vi "cursor window logic -- no plot.vi"(4 "h. offset":dbl, 6 "CursIdx":i32, 7 "cursor window action":T3=enum."check", 8 "window":dbl=nan, 9 "center":dbl=nan, 10 "cursor window in":refnum<vi>, 11 "cursor window init":T2={"left"=2378.60310421286, "right "=2421.6740576496672, "center"=2421.6740576496672, "window"=2421.6740576496672, "cursors"=[], "relative"=0, "absolute"=0, "fixed vertical offset"=2421.6740576496672, "vertical offset"=2421.6740576496672, "skew"=2421.6740576496672, "default window frac"=2421.6740576496672, "kind"=enum."skewed", "skew.left"=2421.6740576496672, "skew.right"=2421.6740576496672, "Plot ref"=refnum, "wing order"=enum."back"}) -> ()   [LabVIEW 2010]
uses:
  stack action -- control.ctl
  cursor window action.ctl
  cursor winow.ctl
  cursor winow control -- no plot.ctl
panel:
  out "cursor window out":T1={"left"=2378.60310421286, "right "=2421.6740576496672, "center"=2421.6740576496672, "window"=2421.6740576496672, "skew"=2421.6740576496672, "default window frac"=2421.6740576496672, "kind"=enum."skewed", "skew.left"=2421.6740576496672, "skew.right"=2421.6740576496672, "wing order"=enum."back"}
  in  "cursor window":T1={"left"=2378.60310421286, "right "=2421.6740576496672, "center"=2421.6740576496672, "window"=2421.6740576496672, "skew"=2421.6740576496672, "default window frac"=2421.6740576496672, "kind"=enum."skewed", "skew.left"=2421.6740576496672, "skew.right"=2421.6740576496672, "wing order"=enum."back"}
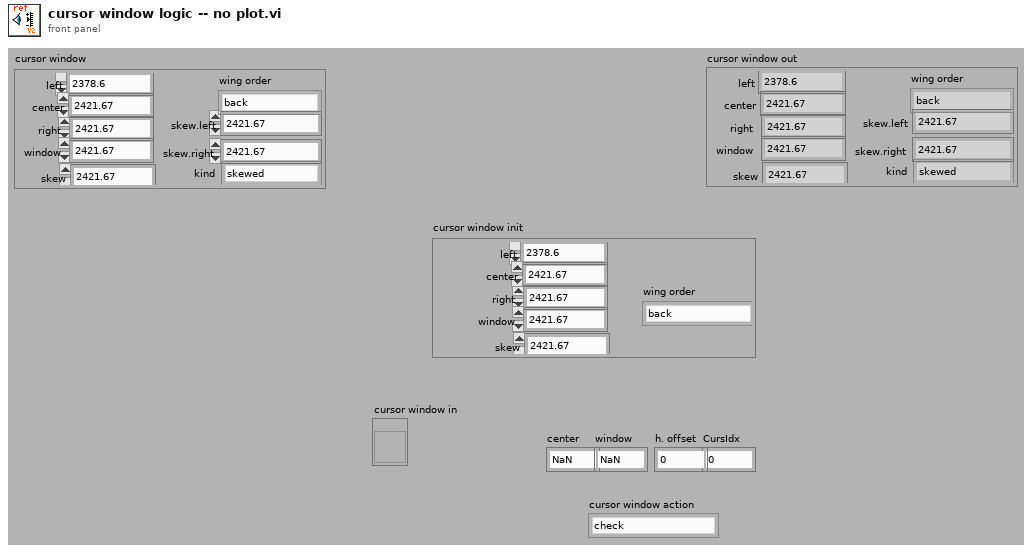
[diagram p1: front panel]
types:
  T1 = typedef "cursor winow control -- no plot.ctl" = cluster{"left":dbl, "right ":dbl, "center":dbl, "window":dbl, "skew":dbl, "default window frac":dbl, "kind":enum16{"symmetric", "skewed", "fancy"}, "skew.left":dbl, "skew.right":dbl, "wing order":enum16{"forw", "back"}}
  T2 = typedef "cursor winow.ctl" = cluster{"left":dbl, "right ":dbl, "center":dbl, "window":dbl, "cursors":i32[], "relative":i32, "absolute":i32, "fixed vertical offset":dbl, "vertical offset":dbl, "skew":dbl, "default window frac":dbl, "kind":enum16{"symmetric", "skewed", "fancy"}, "skew.left":dbl, "skew.right":dbl, "Plot ref":refnum<vi>, "wing order":enum16{"forw", "back"}}
  T3 = typedef "cursor window action.ctl" = enum16{"balance", "h. offset change", "cursor moves", "change center", "change window", "init", "check", "reset", "set y to middle", "idle", "-write all Y", "-write left.X", "-write center.X", "-write right.X", "-write all X", "-change center", "-change window", "-change skew", "-read cursor 2", "-read cursor 1", "-read cursor 0", "-read all cursors", "-reset", "-read plot scale", "-set y to middle", "-Q: center.Y is visible", "-Q: window is visible", "-parse center.Y", "-right left from center", "-left move", "-right move", "-set center.Y", "-empty", "-set cursors to default", "-check", "-write center.Y", "-copy cursor 1", "-copy cursor 0", "-copy cursor 2", "move right", "move left", "shrink", "broaden", "skew up", "skew down", "-write plot scale", "zoom X", "change cen&win"}
  T4 = typedef "stack action -- control.ctl" = enum16{"push", "pop", "check"}
  T5 = cluster{"center":dbl, "window":dbl, "h.offset":dbl, "cursor window":T2}
  T6 = cluster{"right.Y":dbl, "right.X":dbl, "left.X":dbl, "left.Y":dbl, "center.X":dbl, "center.Y":dbl, "scale.x.max":dbl, "scale.x.min":dbl, "scale.y.range":dbl, "scale.y.min":dbl, "scale.x.range":dbl, "scale.y.max":dbl, "skew":dbl, "cursor":i32, "scale.x.center":dbl, "scale.x.halfwidth":dbl, "scale.y.center":dbl, "scale.y.halfwidth":dbl}
  T7 = cluster{"left":dbl, "right ":dbl, "center":dbl, "window":dbl, "cursors":i32[], "relative":i32, "absolute":i32, "fixed vertical offset":dbl, "vertical offset":dbl, "skew":dbl, "default window frac":dbl, "kind":enum16{"symmetric", "skewed", "fancy"}, "skew.left":dbl, "skew.right":dbl, "Plot ref":refnum<vi>, "wing order":enum16{"forw", "back"}}
  T8 = typedef "comparison control.ctl" = enum16{"not a number", "above", "in range", "below"}
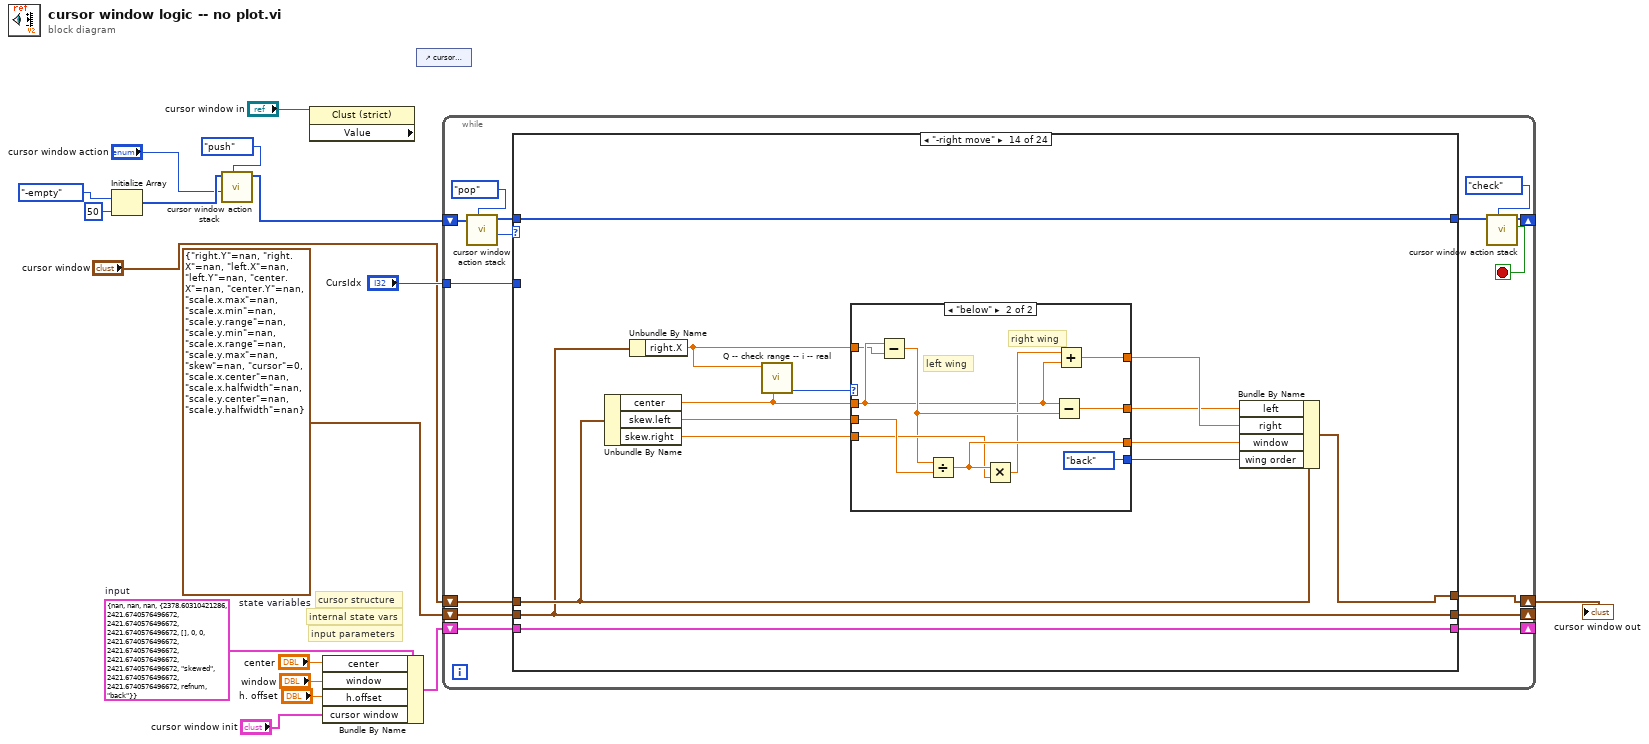
[diagram p0: block diagram]
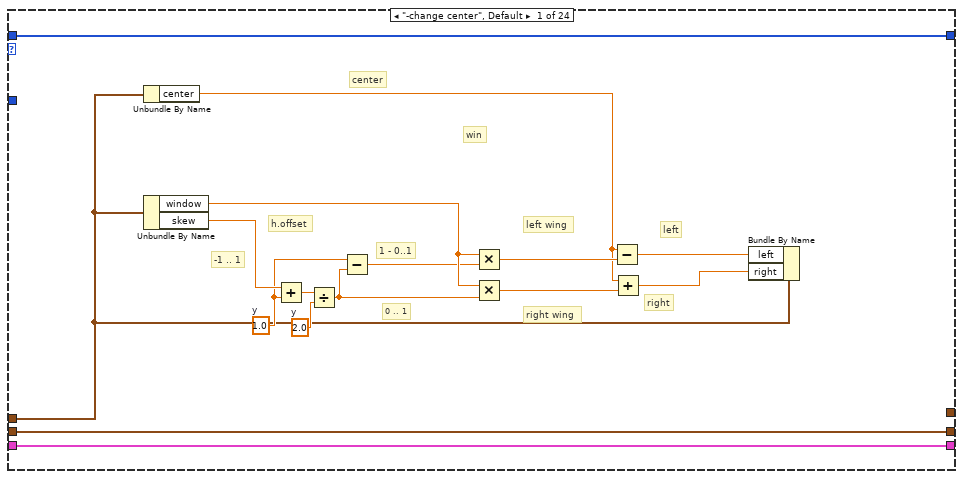
[diagram p2: hidden frame]
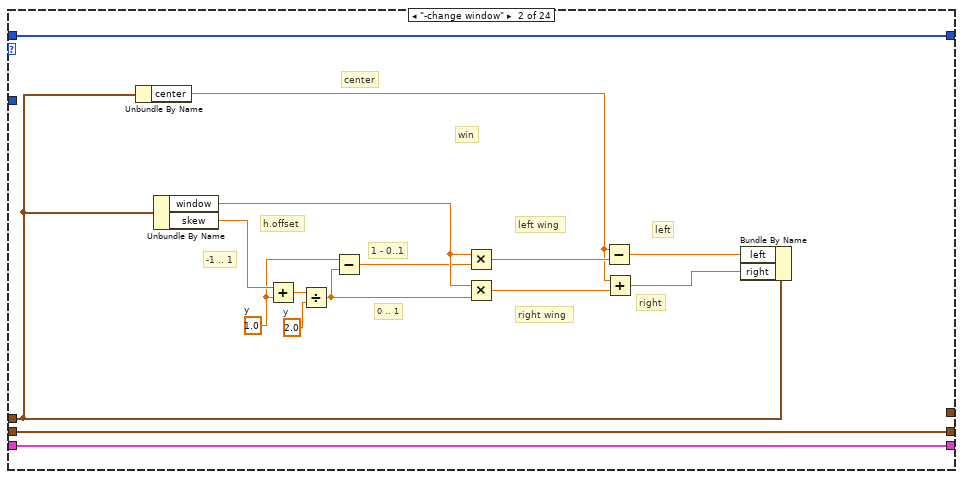
[diagram p3: hidden frame]
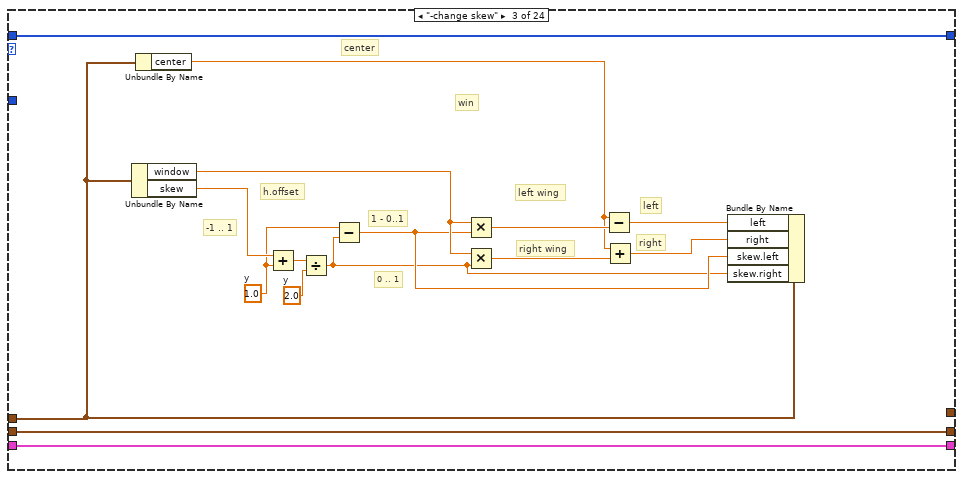
[diagram p4: hidden frame]
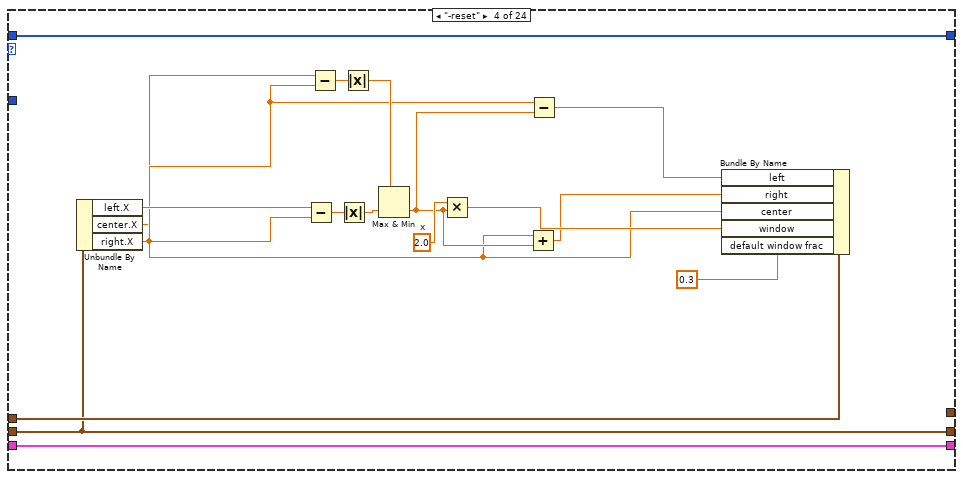
[diagram p5: hidden frame]
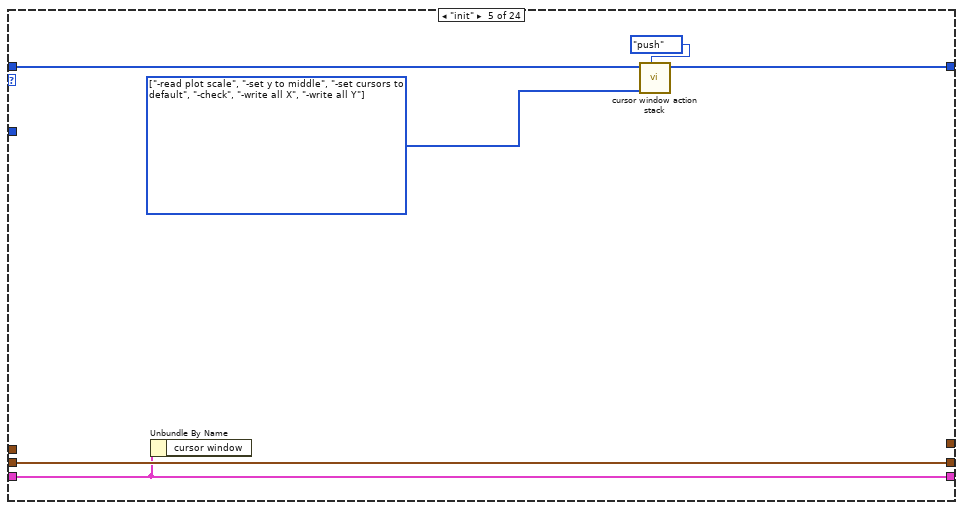
[diagram p6: hidden frame]
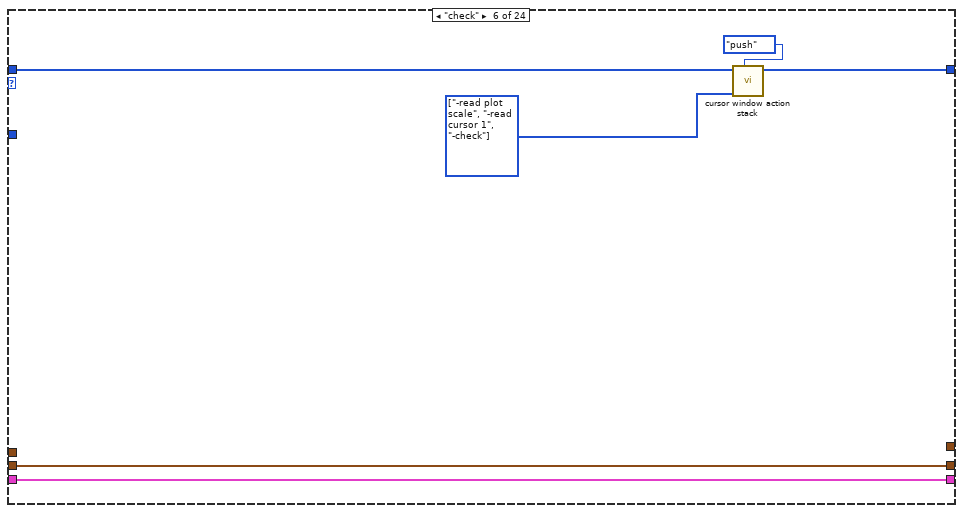
[diagram p7: hidden frame]
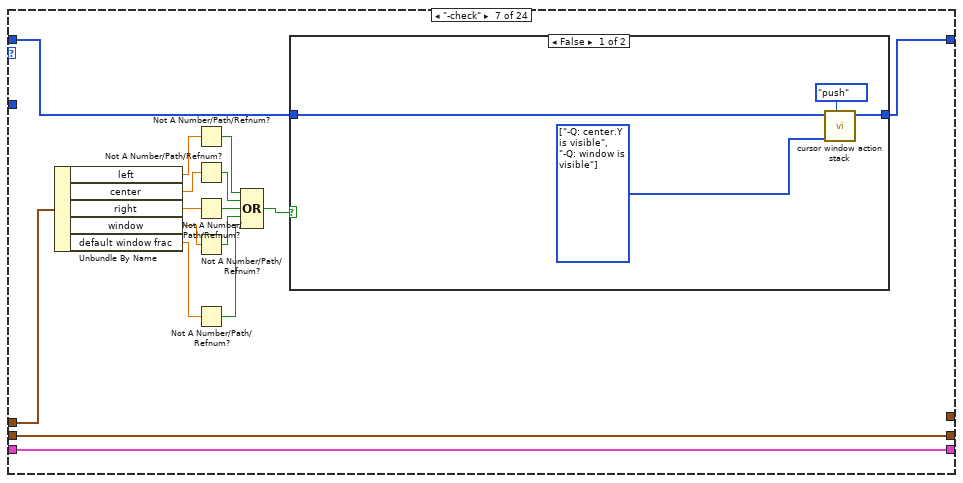
[diagram p8: hidden frame]
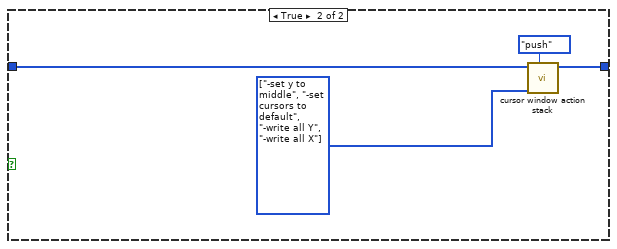
[diagram p9: hidden frame]
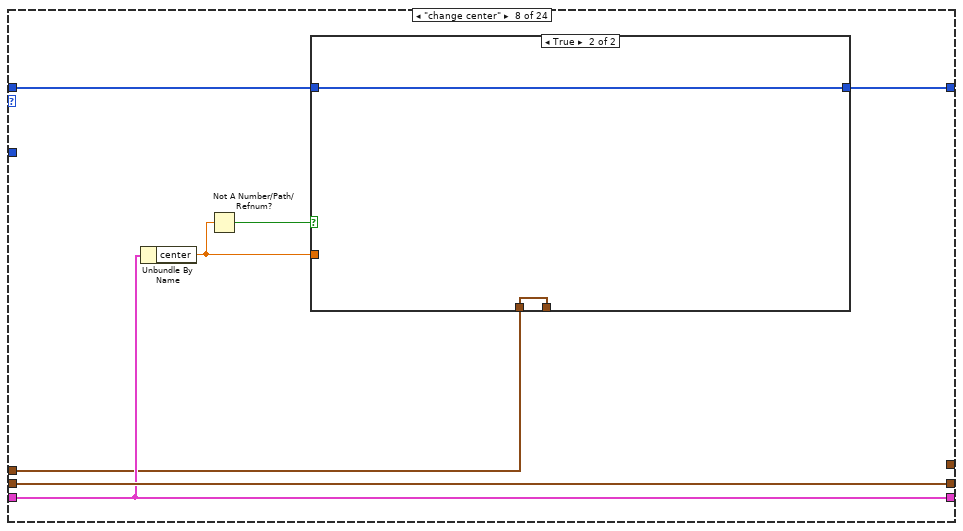
[diagram p10: hidden frame]
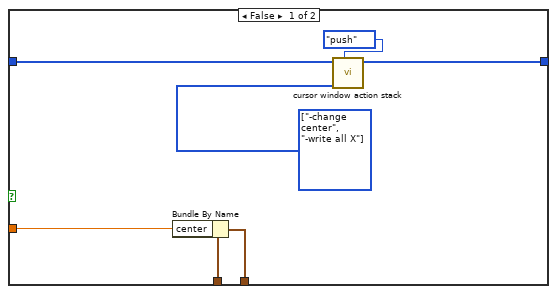
[diagram p11: hidden frame]
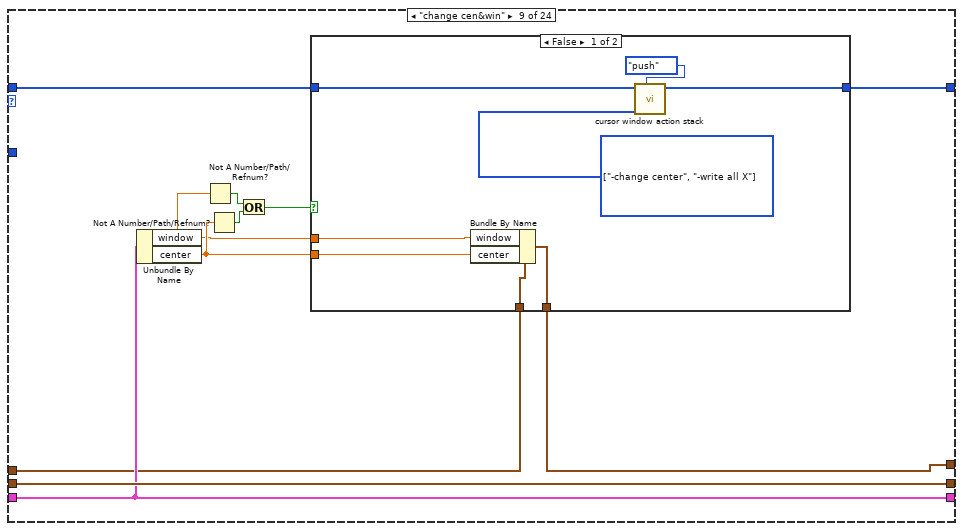
[diagram p12: hidden frame]
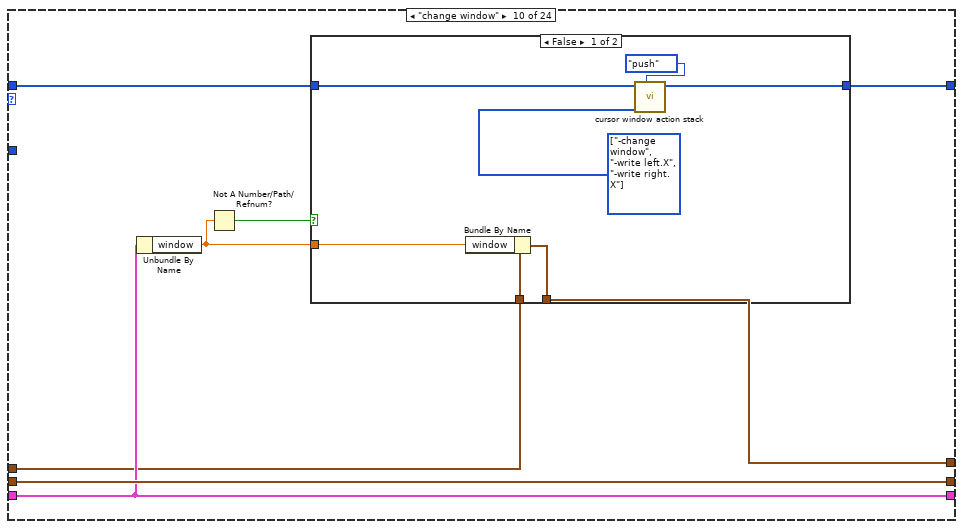
[diagram p14: hidden frame]
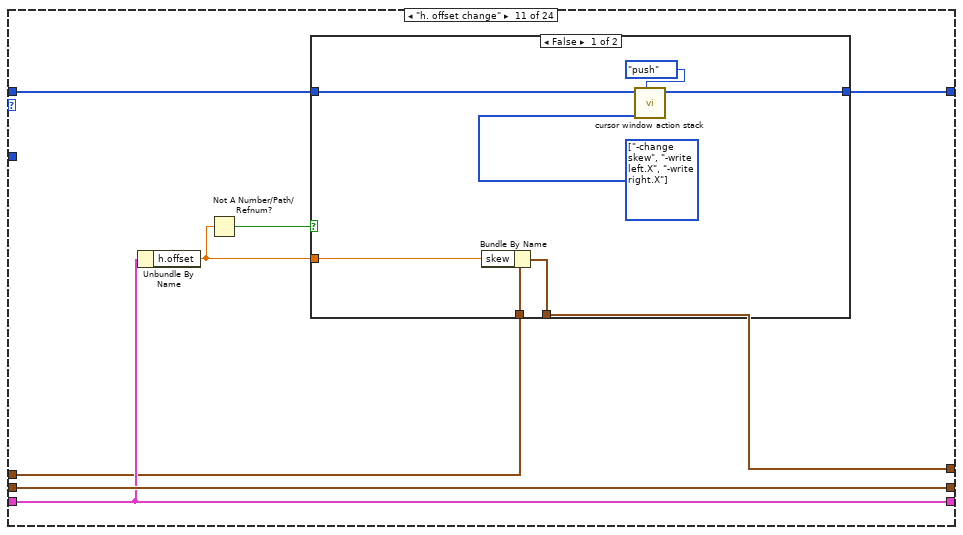
[diagram p16: hidden frame]
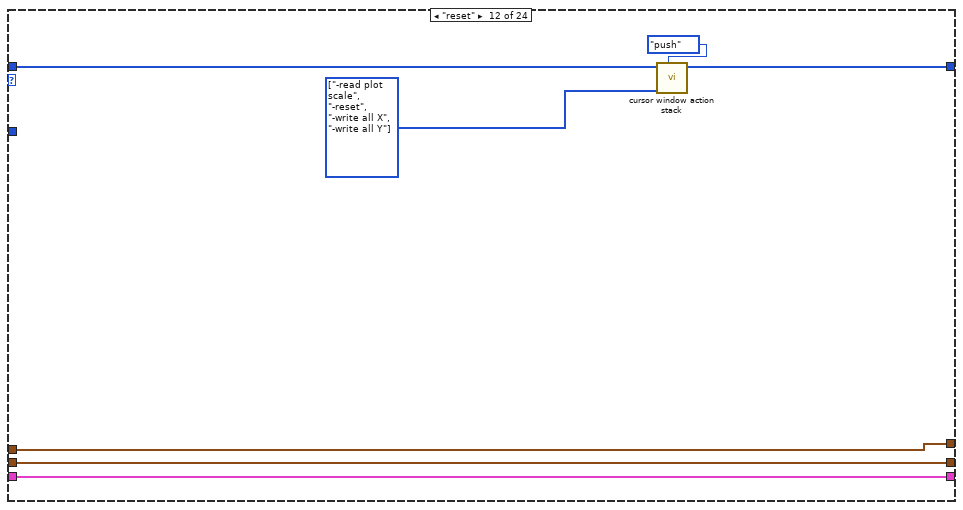
[diagram p18: hidden frame]
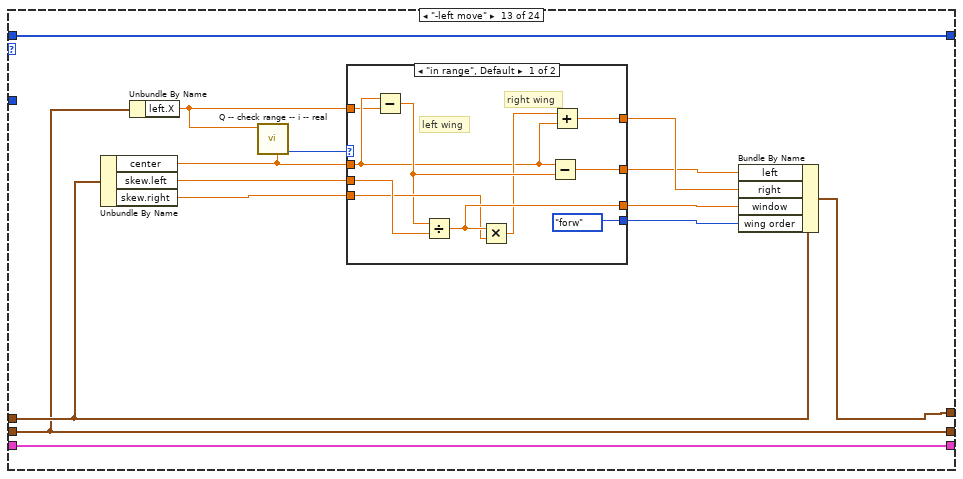
[diagram p19: hidden frame]
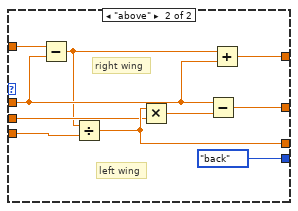
[diagram p20: hidden frame]
diagram:
  w17 = T5 {"center"=nan, "window"=nan, "h.offset"=nan, "cursor window"={"left"=2378.60310421286, "right "=2421.6740576496672, "center"=2421.6740576496672, "window"=2421.6740576496672, "cursors"=[], "relative"=0, "absolute"=0, "fixed vertical offset"=2421.6740576496672, "vertical offset"=2421.6740576496672, "skew"=2421.6740576496672, "default window frac"=2421.6740576496672, "kind"=enum."skewed", "skew.left"=2421.6740576496672, "skew.right"=2421.6740576496672, "Plot ref"=refnum, "wing order"=enum."back"}}  # input
  w18 = T6 {"right.Y"=nan, "right.X"=nan, "left.X"=nan, "left.Y"=nan, "center.X"=nan, "center.Y"=nan, "scale.x.max"=nan, "scale.x.min"=nan, "scale.y.range"=nan, "scale.y.min"=nan, "scale.x.range"=nan, "scale.y.max"=nan, "skew"=nan, "cursor"=0, "scale.x.center"=nan, "scale.x.halfwidth"=nan, "scale.y.center"=nan, "scale.y.halfwidth"=nan}  # state variables
  # "input parameters"
  # "internal state vars"
  # "cursor structure"
  n1 = Initialize Array(cursor_window_action."-empty" ("cursor window action"), 50 ("dimension size")) -> (w6:T3[])
  n2 = call "cursor window action stack.vi"("stack action"=stack_action_--_control."push", "cursor window action"="cursor window action", "command stack"=w6) -> ("command stack out"=w5:T3[])  [unwired: 6 in, 2 out]
  n3 = property class="Clust (strict)"(reference="cursor window in") -> (reference out=w19:refnum<vi>, "Value"=w11:T7)  [unwired: 1 in, 1 out]
  n4 = Bundle By Name(cluster=w17, "center"="center", "window"="window", "h.offset"="h. offset", "cursor window"="cursor window init") -> (w13:T5)
  n5 = control-ref of="cursor window init"() -> ()  [unwired: 1 out]
  n6 = while {
    shift-right: [w27] -> _
    shift-left: w5 -> [w33]
    shift-right: [w20] -> w1
    shift-left: "cursor window" -> [w34]
    shift-right: [w24] -> _
    shift-left: w13 -> [w25]
    shift-right: [w22] -> _
    shift-left: w18 -> [w23]
    tunnel: "CursIdx" -> [w21]
    stop <- w26 stop-if-true
    n7 = call "cursor window action stack.vi"("stack action"=stack_action_--_control."pop", "command stack"=w33) -> ("cursor window action out"=w32:T3, "command stack out"=w30:T3[])  [unwired: 7 in, 1 out]
    n8 = case shown="\"-right move\"" w32 {
      tunnel: w34 -> [w36 w53 w72 w94 _ w111 w121 w143 w164 w181 w198 w214 w231 w265 w291 w302 w315 w329 w335 w355 w361 w374 w395 w419]
      tunnel: [w40 w57 w76 w93 w105 w114 w118 w148 w168 w186 w203 w217 w228 w262 w292 w300 w320 w330 w343 w356 w370 w378 w399 w421] -> w28
      tunnel: w30 -> [w40 w57 w76 w93 w106 w115 w119 w147 w167 w185 w202 w218 w228 w262 w292 w300 w320 w331 w344 w357 w371 w379 w400 w422]
      tunnel: w25 -> [w37 w54 w73 w92 w109 w112 w122 w146 w166 w184 w201 w220 w230 w264 w289 w303 w319 w325 w341 w351 w368 w375 w396 w426]
      tunnel: [w37 w54 w73 w92 w109 w112 w122 w146 w166 w184 w201 w220 w230 w264 w289 w303 w319 w325 w341 w351 w368 w375 w396 w426] -> w24
      tunnel: w23 -> [w39 w56 w75 w91 w110 w113 w123 w149 w169 w187 w204 w219 w229 w263 w290 w305 w318 w326 w342 w352 w369 w376 w397 w425]
      tunnel: [w39 w56 w75 w91 w110 w113 w123 w149 w169 w187 w204 w219 w229 w263 w290 w305 w318 w326 w342 w352 w369 w376 w397 w425] -> w22
      tunnel: w21 -> [_ _ _ _ _ _ _ _ _ _ _ _ _ _ _ _ _ _ _ _ _ _ _ _]
      tunnel: [_ _ _ _ _ _ _ _ w159 w180 w197 w214 w221 w255 _ _ _ _ _ _ _ _ _ _] -> w20
      frame "-change center", Default {
        w45 = 1.0  # y
        w47 = 2.0  # y
        # "1 - 0..1"
        # "right"
        # "left"
        # "win"
        # "h.offset"
        # "center"
        # "left wing"
        # "right wing"
        # "0 .. 1"
        # "-1 .. 1"
        n9 = Unbundle By Name(w36) -> ("center"=w38:dbl)
        n10 = Unbundle By Name(w36) -> ("window"=w50:dbl, "skew"=w51:dbl)
        n11 = Add(x=w51, y=w45) -> (x+y=w46:dbl)
        n12 = Divide(x=w46, y=w47) -> (x/y=w42:dbl)
        n13 = Subtract(x=w45, y=w42) -> (x-y=w41:dbl)
        n14 = Multiply(x=w50, y=w41) -> (x*y=w44:dbl)
        n15 = Multiply(x=w50, y=w42) -> (x*y=w43:dbl)
        n16 = Subtract(x=w38, y=w44) -> (x-y=w49:dbl)
        n17 = Add(x=w38, y=w43) -> (x+y=w48:dbl)
        n18 = Bundle By Name(cluster=w36, "left"=w49, "right"=w48) -> (w35:T1)
      }
      frame "-change window" {
        w62 = 1.0  # y
        w64 = 2.0  # y
        # "1 - 0..1"
        # "right"
        # "left"
        # "win"
        # "h.offset"
        # "center"
        # "left wing"
        # "right wing"
        # "0 .. 1"
        # "-1 .. 1"
        n19 = Unbundle By Name(w53) -> ("center"=w55:dbl)
        n20 = Unbundle By Name(w53) -> ("window"=w67:dbl, "skew"=w68:dbl)
        n21 = Add(x=w68, y=w62) -> (x+y=w63:dbl)
        n22 = Divide(x=w63, y=w64) -> (x/y=w59:dbl)
        n23 = Subtract(x=w62, y=w59) -> (x-y=w58:dbl)
        n24 = Multiply(x=w67, y=w58) -> (x*y=w61:dbl)
        n25 = Multiply(x=w67, y=w59) -> (x*y=w60:dbl)
        n26 = Subtract(x=w55, y=w61) -> (x-y=w66:dbl)
        n27 = Add(x=w55, y=w60) -> (x+y=w65:dbl)
        n28 = Bundle By Name(cluster=w53, "left"=w66, "right"=w65) -> (w52:T1)
      }
      frame "-change skew" {
        w79 = 1.0  # y
        w81 = 2.0  # y
        # "1 - 0..1"
        # "right"
        # "left"
        # "win"
        # "h.offset"
        # "center"
        # "left wing"
        # "right wing"
        # "0 .. 1"
        # "-1 .. 1"
        n29 = Unbundle By Name(w72) -> ("window"=w84:dbl, "skew"=w85:dbl)
        n30 = Unbundle By Name(w72) -> ("center"=w74:dbl)
        n31 = Add(x=w85, y=w79) -> (x+y=w80:dbl)
        n32 = Divide(x=w80, y=w81) -> (x/y=w70:dbl)
        n33 = Subtract(x=w79, y=w70) -> (x-y=w71:dbl)
        n34 = Multiply(x=w84, y=w71) -> (x*y=w78:dbl)
        n35 = Multiply(x=w84, y=w70) -> (x*y=w77:dbl)
        n36 = Subtract(x=w74, y=w78) -> (x-y=w83:dbl)
        n37 = Add(x=w74, y=w77) -> (x+y=w82:dbl)
        n38 = Bundle By Name(cluster=w72, "left"=w83, "right"=w82, "skew.left"=w71, "skew.right"=w70) -> (w69:T1)
      }
      frame "-reset" {
        w99 = 2.0  # x
        n39 = Unbundle By Name(w91) -> ("left.X"=w90:dbl, "center.X"=w88:dbl, "right.X"=w89:dbl)
        n40 = Subtract(x=w90, y=w89) -> (x-y=w102:dbl)
        n41 = Subtract(x=w88, y=w89) -> (x-y=w103:dbl)
        n42 = Absolute Value(x=w102) -> (abs(x)=w100:dbl)
        n43 = Absolute Value(x=w103) -> (abs(x)=w101:dbl)
        n44 = Max & Min(x=w101, y=w100) -> (min(x,y)=w97:dbl)  [unwired: 1 out]
        n45 = Multiply(x=w99, y=w97) -> (x*y=w98:dbl)
        n46 = Add(x=w89, y=w97) -> (x+y=w95:dbl)
        n47 = Subtract(x=w89, y=w97) -> (x-y=w96:dbl)
        n48 = Bundle By Name(cluster=w94, "left"=w96, "right"=w95, "center"=w89, "window"=w98, "default window frac"=0.3) -> (w87:T1)
      }
      frame "init" {
        w107 = T3[] [enum."-read plot scale", enum."-set y to middle", enum."-set cursors to default", enum."-check", enum."-write all X", enum."-write all Y"] items=["balance", "h. offset change", "cursor moves", "change center", "change window", "init", "check", "reset", "set y to middle", "idle", "-write all Y", "-write left.X", "-write center.X", "-write right.X", "-write all X", "-change center", "-change window", "-change skew", "-read cursor 2", "-read cursor 1", "-read cursor 0", "-read all cursors", "-reset", "-read plot scale", "-set y to middle", "-Q: center.Y is visible", "-Q: window is visible", "-parse center.Y", "-right left from center", "-left move", "-right move", "-set center.Y", "-empty", "-set cursors to default", "-check", "-write center.Y", "-copy cursor 1", "-copy cursor 0", "-copy cursor 2", "move right", "move left", "shrink", "broaden", "skew up", "skew down", "-write plot scale", "zoom X", "change cen&win"]
        n49 = Unbundle By Name(w109) -> ("cursor window"=w104:T2)
        n50 = call "cursor window action stack.vi"("stack action"=stack_action_--_control."push", "action list"=w107, "command stack"=w106) -> ("command stack out"=w105:T3[])  [unwired: 6 in, 2 out]
      }
      frame "check" {
        w116 = T3[] [enum."-read plot scale", enum."-read cursor 1", enum."-check"] items=["balance", "h. offset change", "cursor moves", "change center", "change window", "init", "check", "reset", "set y to middle", "idle", "-write all Y", "-write left.X", "-write center.X", "-write right.X", "-write all X", "-change center", "-change window", "-change skew", "-read cursor 2", "-read cursor 1", "-read cursor 0", "-read all cursors", "-reset", "-read plot scale", "-set y to middle", "-Q: center.Y is visible", "-Q: window is visible", "-parse center.Y", "-right left from center", "-left move", "-right move", "-set center.Y", "-empty", "-set cursors to default", "-check", "-write center.Y", "-copy cursor 1", "-copy cursor 0", "-copy cursor 2", "move right", "move left", "shrink", "broaden", "skew up", "skew down", "-write plot scale", "zoom X", "change cen&win"]
        n51 = call "cursor window action stack.vi"("stack action"=stack_action_--_control."push", "action list"=w116, "command stack"=w115) -> ("command stack out"=w114:T3[])  [unwired: 6 in, 2 out]
      }
      frame "-check" {
        n52 = Unbundle By Name(w121) -> ("left"=w131:dbl, "center"=w130:dbl, "right"=w132:dbl, "window"=w133:dbl, "default window frac"=w125:dbl)
        n53 = Not A Number/Path/Refnum?(number/path/refnum=w131) -> (NaN/Path/Refnum?=w129:bool)
        n54 = Not A Number/Path/Refnum?(number/path/refnum=w130) -> (NaN/Path/Refnum?=w128:bool)
        n55 = Not A Number/Path/Refnum?(number/path/refnum=w132) -> (NaN/Path/Refnum?=w127:bool)
        n56 = Not A Number/Path/Refnum?(number/path/refnum=w133) -> (NaN/Path/Refnum?=w126:bool)
        n57 = Not A Number/Path/Refnum?(number/path/refnum=w125) -> (NaN/Path/Refnum?=w124:bool)
        n58 = Compound Arithmetic op=OR(w129, w128, w127, w126, w124) -> (w120:bool)
        n59 = case shown="False" w120 {
          tunnel: w119 -> [w135 w139]
          tunnel: [w134 w138] -> w118
          frame False {
            w136 = T3[] [enum."-Q: center.Y is visible", enum."-Q: window is visible"] items=["balance", "h. offset change", "cursor moves", "change center", "change window", "init", "check", "reset", "set y to middle", "idle", "-write all Y", "-write left.X", "-write center.X", "-write right.X", "-write all X", "-change center", "-change window", "-change skew", "-read cursor 2", "-read cursor 1", "-read cursor 0", "-read all cursors", "-reset", "-read plot scale", "-set y to middle", "-Q: center.Y is visible", "-Q: window is visible", "-parse center.Y", "-right left from center", "-left move", "-right move", "-set center.Y", "-empty", "-set cursors to default", "-check", "-write center.Y", "-copy cursor 1", "-copy cursor 0", "-copy cursor 2", "move right", "move left", "shrink", "broaden", "skew up", "skew down", "-write plot scale", "zoom X", "change cen&win"]
            n60 = call "cursor window action stack.vi"("stack action"=stack_action_--_control."push", "action list"=w136, "command stack"=w135) -> ("command stack out"=w134:T3[])  [unwired: 6 in, 2 out]
          }
          frame True {
            w140 = T3[] [enum."-set y to middle", enum."-set cursors to default", enum."-write all Y", enum."-write all X"] items=["balance", "h. offset change", "cursor moves", "change center", "change window", "init", "check", "reset", "set y to middle", "idle", "-write all Y", "-write left.X", "-write center.X", "-write right.X", "-write all X", "-change center", "-change window", "-change skew", "-read cursor 2", "-read cursor 1", "-read cursor 0", "-read all cursors", "-reset", "-read plot scale", "-set y to middle", "-Q: center.Y is visible", "-Q: window is visible", "-parse center.Y", "-right left from center", "-left move", "-right move", "-set center.Y", "-empty", "-set cursors to default", "-check", "-write center.Y", "-copy cursor 1", "-copy cursor 0", "-copy cursor 2", "move right", "move left", "shrink", "broaden", "skew up", "skew down", "-write plot scale", "zoom X", "change cen&win"]
            n61 = call "cursor window action stack.vi"("stack action"=stack_action_--_control."push", "action list"=w140, "command stack"=w139) -> ("command stack out"=w138:T3[])  [unwired: 6 in, 2 out]
          }
        }
      }
      frame "change center" {
        n62 = Unbundle By Name(w146) -> ("center"=w144:dbl)
        n63 = Not A Number/Path/Refnum?(number/path/refnum=w144) -> (NaN/Path/Refnum?=w145:bool)
        n64 = case shown="True" w145 {
          tunnel: [w156 w157] -> w148
          tunnel: w147 -> [w155 w157]
          tunnel: w143 -> [w152 w158]
          tunnel: w144 -> [w151 _]
          tunnel: [w150 w158] -> w142
          frame False {
            w153 = T3[] [enum."-change center", enum."-write all X"] items=["balance", "h. offset change", "cursor moves", "change center", "change window", "init", "check", "reset", "set y to middle", "idle", "-write all Y", "-write left.X", "-write center.X", "-write right.X", "-write all X", "-change center", "-change window", "-change skew", "-read cursor 2", "-read cursor 1", "-read cursor 0", "-read all cursors", "-reset", "-read plot scale", "-set y to middle", "-Q: center.Y is visible", "-Q: window is visible", "-parse center.Y", "-right left from center", "-left move", "-right move", "-set center.Y", "-empty", "-set cursors to default", "-check", "-write center.Y", "-copy cursor 1", "-copy cursor 0", "-copy cursor 2", "move right", "move left", "shrink", "broaden", "skew up", "skew down", "-write plot scale", "zoom X", "change cen&win"]
            n65 = Bundle By Name(cluster=w152, "center"=w151) -> (w150:T1)
            n66 = call "cursor window action stack.vi"("stack action"=stack_action_--_control."push", "action list"=w153, "command stack"=w155) -> ("command stack out"=w156:T3[])  [unwired: 6 in, 2 out]
          }
          frame True {
          }
        }
      }
      frame "change cen&win" {
        n67 = Unbundle By Name(w166) -> ("window"=w160:dbl, "center"=w165:dbl)
        n68 = Not A Number/Path/Refnum?(number/path/refnum=w160) -> (NaN/Path/Refnum?=w163:bool)
        n69 = Not A Number/Path/Refnum?(number/path/refnum=w165) -> (NaN/Path/Refnum?=w162:bool)
        n70 = Or(x=w163, y=w162) -> (x .or. y?=w161:bool)
        n71 = case shown="False" w161 {
          tunnel: [w177 w178] -> w168
          tunnel: w167 -> [w176 w178]
          tunnel: w164 -> [w173 w179]
          tunnel: w165 -> [w172 _]
          tunnel: [w171 w179] -> w159
          tunnel: w160 -> [w170 _]
          frame False {
            w174 = T3[] [enum."-change center", enum."-write all X"] items=["balance", "h. offset change", "cursor moves", "change center", "change window", "init", "check", "reset", "set y to middle", "idle", "-write all Y", "-write left.X", "-write center.X", "-write right.X", "-write all X", "-change center", "-change window", "-change skew", "-read cursor 2", "-read cursor 1", "-read cursor 0", "-read all cursors", "-reset", "-read plot scale", "-set y to middle", "-Q: center.Y is visible", "-Q: window is visible", "-parse center.Y", "-right left from center", "-left move", "-right move", "-set center.Y", "-empty", "-set cursors to default", "-check", "-write center.Y", "-copy cursor 1", "-copy cursor 0", "-copy cursor 2", "move right", "move left", "shrink", "broaden", "skew up", "skew down", "-write plot scale", "zoom X", "change cen&win"]
            n72 = Bundle By Name(cluster=w173, "window"=w170, "center"=w172) -> (w171:T1)
            n73 = call "cursor window action stack.vi"("stack action"=stack_action_--_control."push", "action list"=w174, "command stack"=w176) -> ("command stack out"=w177:T3[])  [unwired: 6 in, 2 out]
          }
          frame True {
          }
        }
      }
      frame "change window" {
        n74 = Unbundle By Name(w184) -> ("window"=w182:dbl)
        n75 = Not A Number/Path/Refnum?(number/path/refnum=w182) -> (NaN/Path/Refnum?=w183:bool)
        n76 = case shown="False" w183 {
          tunnel: [w194 w195] -> w186
          tunnel: w185 -> [w193 w195]
          tunnel: w181 -> [w190 w196]
          tunnel: w182 -> [w189 _]
          tunnel: [w188 w196] -> w180
          frame False {
            w191 = T3[] [enum."-change window", enum."-write left.X", enum."-write right.X"] items=["balance", "h. offset change", "cursor moves", "change center", "change window", "init", "check", "reset", "set y to middle", "idle", "-write all Y", "-write left.X", "-write center.X", "-write right.X", "-write all X", "-change center", "-change window", "-change skew", "-read cursor 2", "-read cursor 1", "-read cursor 0", "-read all cursors", "-reset", "-read plot scale", "-set y to middle", "-Q: center.Y is visible", "-Q: window is visible", "-parse center.Y", "-right left from center", "-left move", "-right move", "-set center.Y", "-empty", "-set cursors to default", "-check", "-write center.Y", "-copy cursor 1", "-copy cursor 0", "-copy cursor 2", "move right", "move left", "shrink", "broaden", "skew up", "skew down", "-write plot scale", "zoom X", "change cen&win"]
            n77 = Bundle By Name(cluster=w190, "window"=w189) -> (w188:T1)
            n78 = call "cursor window action stack.vi"("stack action"=stack_action_--_control."push", "action list"=w191, "command stack"=w193) -> ("command stack out"=w194:T3[])  [unwired: 6 in, 2 out]
          }
          frame True {
          }
        }
      }
      frame "h. offset change" {
        n79 = Unbundle By Name(w201) -> ("h.offset"=w199:dbl)
        n80 = Not A Number/Path/Refnum?(number/path/refnum=w199) -> (NaN/Path/Refnum?=w200:bool)
        n81 = case shown="False" w200 {
          tunnel: [w211 w212] -> w203
          tunnel: w202 -> [w210 w212]
          tunnel: w198 -> [w207 w213]
          tunnel: w199 -> [w206 _]
          tunnel: [w205 w213] -> w197
          frame False {
            w208 = T3[] [enum."-change skew", enum."-write left.X", enum."-write right.X"] items=["balance", "h. offset change", "cursor moves", "change center", "change window", "init", "check", "reset", "set y to middle", "idle", "-write all Y", "-write left.X", "-write center.X", "-write right.X", "-write all X", "-change center", "-change window", "-change skew", "-read cursor 2", "-read cursor 1", "-read cursor 0", "-read all cursors", "-reset", "-read plot scale", "-set y to middle", "-Q: center.Y is visible", "-Q: window is visible", "-parse center.Y", "-right left from center", "-left move", "-right move", "-set center.Y", "-empty", "-set cursors to default", "-check", "-write center.Y", "-copy cursor 1", "-copy cursor 0", "-copy cursor 2", "move right", "move left", "shrink", "broaden", "skew up", "skew down", "-write plot scale", "zoom X", "change cen&win"]
            n82 = Bundle By Name(cluster=w207, "skew"=w206) -> (w205:T1)
            n83 = call "cursor window action stack.vi"("stack action"=stack_action_--_control."push", "action list"=w208, "command stack"=w210) -> ("command stack out"=w211:T3[])  [unwired: 6 in, 2 out]
          }
          frame True {
          }
        }
      }
      frame "reset" {
        w215 = T3[] [enum."-read plot scale", enum."-reset", enum."-write all X", enum."-write all Y"] items=["balance", "h. offset change", "cursor moves", "change center", "change window", "init", "check", "reset", "set y to middle", "idle", "-write all Y", "-write left.X", "-write center.X", "-write right.X", "-write all X", "-change center", "-change window", "-change skew", "-read cursor 2", "-read cursor 1", "-read cursor 0", "-read all cursors", "-reset", "-read plot scale", "-set y to middle", "-Q: center.Y is visible", "-Q: window is visible", "-parse center.Y", "-right left from center", "-left move", "-right move", "-set center.Y", "-empty", "-set cursors to default", "-check", "-write center.Y", "-copy cursor 1", "-copy cursor 0", "-copy cursor 2", "move right", "move left", "shrink", "broaden", "skew up", "skew down", "-write plot scale", "zoom X", "change cen&win"]
        n84 = call "cursor window action stack.vi"("stack action"=stack_action_--_control."push", "action list"=w215, "command stack"=w218) -> ("command stack out"=w217:T3[])  [unwired: 6 in, 2 out]
      }
      frame "-left move" {
        n85 = Unbundle By Name(w231) -> ("center"=w224:dbl, "skew.left"=w227:dbl, "skew.right"=w226:dbl)
        n86 = Unbundle By Name(w229) -> ("left.X"=w225:dbl)
        n87 = call "Q -- check range -- i -- real.vi"("upper"=w224, "number"=w225) -> ("selector"=w223:T8)  [unwired: 7 in, 2 out]
        n88 = case shown="\"in range\", Default" w223 {
          tunnel: w225 -> [w236 w254]
          tunnel: w226 -> [w242 w253]
          tunnel: [w243 w252] -> w232
          tunnel: [w238 w247] -> w234
          tunnel: w227 -> [w244 w251]
          tunnel: [w240 w246] -> w233
          tunnel: w224 -> [w237 w250]
          tunnel: [enum16{"forw", "back"}."forw" ("wing order") enum16{"forw", "back"}."back" ("wing order")] -> w222
          frame "in range", Default {
            # "right wing"
            # "left wing"
            n89 = Subtract(x=w237, y=w236) -> (x-y=w241:dbl)
            n90 = Divide(x=w241, y=w244) -> (x/y=w243:dbl)
            n91 = Multiply(x=w243, y=w242) -> (x*y=w239:dbl)
            n92 = Subtract(x=w237, y=w241) -> (x-y=w240:dbl)
            n93 = Add(x=w239, y=w237) -> (x+y=w238:dbl)
          }
          frame "above" {
            # "right wing"
            # "left wing"
            n94 = Subtract(x=w254, y=w250) -> (x-y=w249:dbl)
            n95 = Divide(x=w249, y=w253) -> (x/y=w252:dbl)
            n96 = Multiply(x=w252, y=w251) -> (x*y=w248:dbl)
            n97 = Subtract(x=w250, y=w248) -> (x-y=w246:dbl)
            n98 = Add(x=w249, y=w250) -> (x+y=w247:dbl)
          }
        }
        n99 = Bundle By Name(cluster=w231, "left"=w233, "right"=w234, "window"=w232, "wing order"=w222) -> (w221:T1)
      }
      frame "-right move" {
        n100 = Unbundle By Name(w265) -> ("center"=w256:dbl, "skew.left"=w261:dbl, "skew.right"=w260:dbl)
        n101 = Unbundle By Name(w263) -> ("right.X"=w259:dbl)
        n102 = call "Q -- check range -- i -- real.vi"("lower"=w256, "number"=w259) -> ("selector"=w258:T8)  [unwired: 7 in, 2 out]
        n103 = case shown="\"below\"" w258 {
          tunnel: w259 -> [w278 w280]
          tunnel: w260 -> [w277 w286]
          tunnel: [w276 w287] -> w266
          tunnel: [w271 w282] -> w268
          tunnel: w261 -> [w275 w288]
          tunnel: [w270 w284] -> w267
          tunnel: w256 -> [w274 w281]
          tunnel: [enum16{"forw", "back"}."forw" ("wing order") enum16{"forw", "back"}."back" ("wing order")] -> w257
          frame "in range", Default {
            # "right wing"
            n104 = Subtract(x=w278, y=w274) -> (x-y=w273:dbl)
            n105 = Divide(x=w273, y=w277) -> (x/y=w276:dbl)
            n106 = Multiply(x=w276, y=w275) -> (x*y=w272:dbl)
            n107 = Subtract(x=w274, y=w272) -> (x-y=w270:dbl)
            n108 = Add(x=w273, y=w274) -> (x+y=w271:dbl)
          }
          frame "below" {
            # "right wing"
            # "left wing"
            n109 = Subtract(x=w281, y=w280) -> (x-y=w285:dbl)
            n110 = Divide(x=w285, y=w288) -> (x/y=w287:dbl)
            n111 = Multiply(x=w287, y=w286) -> (x*y=w283:dbl)
            n112 = Subtract(x=w281, y=w285) -> (x-y=w284:dbl)
            n113 = Add(x=w283, y=w281) -> (x+y=w282:dbl)
          }
        }
        n114 = Bundle By Name(cluster=w265, "left"=w267, "right"=w268, "window"=w266, "wing order"=w257) -> (w255:T1)
      }
      frame "idle" {
        n115 = disable-structure shown="Disabled" {
          frame Disabled {
            w293 = "win:left"  # Name
            w299 = u32 0  # Cursor Mode
            w298 = TRUE  # Allow Drag
            w297 = FALSE  # Name Visible
            w296 = u8 0  # Point Style
            w295 = u8 2  # Style
            n116 = Bundle By Name("Name"=w293, "Color"=u32 16768256, "Style"=w295, "Point Style"=w296, "Name Visible"=w297, "Allow Drag"=w298, "Cursor Mode"=w299) -> ()  [unwired: 1 in, 1 out]
            n117 = call "Q -- check range -- i -- real.vi"() -> ()  [unwired: 9 in, 3 out]
          }
          frame Enabled {
          }
        }
      }
      frame "-copy cursor 1" {
        n118 = Unbundle By Name(w305) -> ("center.X"=w304:dbl)
        n119 = Bundle By Name(cluster=w302, "center"=w304) -> (w301:T1)
      }
      frame "-set cursors to default" {
        w309 = 0.5
        w308 = 0.1
        (unwired) 3
        (unwired) 0.0
        n120 = Unbundle By Name(w318) -> ("scale.x.halfwidth"=w307:dbl, "scale.x.center"=w313:dbl)
        n121 = Multiply(x=w307, y=w308) -> (x*y=w306:dbl)
        n122 = Multiply(x=w306, y=2) -> (x*y=w312:dbl)
        n123 = Add(x=w313, y=w306) -> (x+y=w316:dbl)
        n124 = Subtract(x=w313, y=w306) -> (x-y=w317:dbl)
        n125 = Bundle By Name(cluster=w315, "default window frac"=w308, "left"=w317, "right"=w316, "center"=w313, "window"=w312, "skew"=0.0, "skew.left"=w309, "skew.right"=w309) -> (w311:T1)
      }
      frame "move left" {
        (unwired) 0.2
        w333 = T3[] [enum."-change center", enum."-write all X"] items=["balance", "h. offset change", "cursor moves", "change center", "change window", "init", "check", "reset", "set y to middle", "idle", "-write all Y", "-write left.X", "-write center.X", "-write right.X", "-write all X", "-change center", "-change window", "-change skew", "-read cursor 2", "-read cursor 1", "-read cursor 0", "-read all cursors", "-reset", "-read plot scale", "-set y to middle", "-Q: center.Y is visible", "-Q: window is visible", "-parse center.Y", "-right left from center", "-left move", "-right move", "-set center.Y", "-empty", "-set cursors to default", "-check", "-write center.Y", "-copy cursor 1", "-copy cursor 0", "-copy cursor 2", "move right", "move left", "shrink", "broaden", "skew up", "skew down", "-write plot scale", "zoom X", "change cen&win"]
        n126 = Unbundle By Name(w329) -> ("center"=w323:dbl, "window"=w322:dbl, "default window frac"=w321:dbl)  [unwired: 1 out]
        n127 = Multiply(x=w322, y=w321) -> (x*y=w324:dbl)
        n128 = Subtract(x=w323, y=w324) -> (x-y=w327:dbl)
        n129 = Bundle By Name(cluster=w329, "center"=w327) -> (w328:T1)
        n130 = call "cursor window action stack.vi"("stack action"=stack_action_--_control."push", "action list"=w333, "command stack"=w331) -> ("command stack out"=w330:T3[])  [unwired: 6 in, 2 out]
      }
      frame "move right" {
        (unwired) 0.2
        w346 = T3[] [enum."-change center", enum."-write all X"] items=["balance", "h. offset change", "cursor moves", "change center", "change window", "init", "check", "reset", "set y to middle", "idle", "-write all Y", "-write left.X", "-write center.X", "-write right.X", "-write all X", "-change center", "-change window", "-change skew", "-read cursor 2", "-read cursor 1", "-read cursor 0", "-read all cursors", "-reset", "-read plot scale", "-set y to middle", "-Q: center.Y is visible", "-Q: window is visible", "-parse center.Y", "-right left from center", "-left move", "-right move", "-set center.Y", "-empty", "-set cursors to default", "-check", "-write center.Y", "-copy cursor 1", "-copy cursor 0", "-copy cursor 2", "move right", "move left", "shrink", "broaden", "skew up", "skew down", "-write plot scale", "zoom X", "change cen&win"]
        n131 = Unbundle By Name(w335) -> ("center"=w338:dbl, "window"=w337:dbl, "default window frac"=w336:dbl)  [unwired: 1 out]
        n132 = Multiply(x=w337, y=w336) -> (x*y=w339:dbl)
        n133 = Add(x=w338, y=w339) -> (x+y=w340:dbl)
        n134 = Bundle By Name(cluster=w335, "center"=w340) -> (w334:T1)
        n135 = call "cursor window action stack.vi"("stack action"=stack_action_--_control."push", "action list"=w346, "command stack"=w344) -> ("command stack out"=w343:T3[])  [unwired: 6 in, 2 out]
      }
      frame "shrink" {
        (unwired) 0.3
        w359 = T3[] [enum."-change window", enum."-write all X", enum."-read plot scale", enum."-set center.Y", enum."-write center.Y"] items=["balance", "h. offset change", "cursor moves", "change center", "change window", "init", "check", "reset", "set y to middle", "idle", "-write all Y", "-write left.X", "-write center.X", "-write right.X", "-write all X", "-change center", "-change window", "-change skew", "-read cursor 2", "-read cursor 1", "-read cursor 0", "-read all cursors", "-reset", "-read plot scale", "-set y to middle", "-Q: center.Y is visible", "-Q: window is visible", "-parse center.Y", "-right left from center", "-left move", "-right move", "-set center.Y", "-empty", "-set cursors to default", "-check", "-write center.Y", "-copy cursor 1", "-copy cursor 0", "-copy cursor 2", "move right", "move left", "shrink", "broaden", "skew up", "skew down", "-write plot scale", "zoom X", "change cen&win"]
        n136 = Unbundle By Name(w355) -> ("window"=w350:dbl, "window"=w349:dbl, "default window frac"=w347:dbl)
        n137 = Multiply(x=w349, y=w347) -> (x*y=w348:dbl)
        n138 = Subtract(x=w350, y=w348) -> (x-y=w353:dbl)
        n139 = Bundle By Name(cluster=w355, "window"=w353) -> (w354:T1)
        n140 = call "cursor window action stack.vi"("stack action"=stack_action_--_control."push", "action list"=w359, "command stack"=w357) -> ("command stack out"=w356:T3[])  [unwired: 6 in, 2 out]
      }
      frame "broaden" {
        (unwired) 0.3
        w367 = T3[] [enum."-change window", enum."-write all X", enum."-read plot scale", enum."-set center.Y", enum."-write center.Y"] items=["balance", "h. offset change", "cursor moves", "change center", "change window", "init", "check", "reset", "set y to middle", "idle", "-write all Y", "-write left.X", "-write center.X", "-write right.X", "-write all X", "-change center", "-change window", "-change skew", "-read cursor 2", "-read cursor 1", "-read cursor 0", "-read all cursors", "-reset", "-read plot scale", "-set y to middle", "-Q: center.Y is visible", "-Q: window is visible", "-parse center.Y", "-right left from center", "-left move", "-right move", "-set center.Y", "-empty", "-set cursors to default", "-check", "-write center.Y", "-copy cursor 1", "-copy cursor 0", "-copy cursor 2", "move right", "move left", "shrink", "broaden", "skew up", "skew down", "-write plot scale", "zoom X", "change cen&win"]
        n141 = Unbundle By Name(w361) -> ("window"=w365:dbl, "window"=w364:dbl, "default window frac"=w362:dbl)
        n142 = Multiply(x=w364, y=w362) -> (x*y=w363:dbl)
        n143 = Add(x=w365, y=w363) -> (x+y=w366:dbl)
        n144 = Bundle By Name(cluster=w361, "window"=w366) -> (w360:T1)
        n145 = call "cursor window action stack.vi"("stack action"=stack_action_--_control."push", "action list"=w367, "command stack"=w371) -> ("command stack out"=w370:T3[])  [unwired: 6 in, 2 out]
      }
      frame "skew up" {
        n146 = Unbundle By Name(w374) -> ("kind"=w373:enum16{"symmetric", "skewed", "fancy"})
        n147 = case shown="\"skewed\"" w373 {
          tunnel: w379 -> [w381 w391]
          tunnel: [w381 w390] -> w378
          tunnel: [w380 w389] -> w377
          tunnel: w374 -> [w380 w387]
          frame "symmetric", Default {
          }
          frame "skewed" {
            w393 = T3[] [enum."-change skew", enum."-read plot scale", enum."-set center.Y", enum."-write right.X", enum."-write left.X", enum."-write center.Y"] items=["balance", "h. offset change", "cursor moves", "change center", "change window", "init", "check", "reset", "set y to middle", "idle", "-write all Y", "-write left.X", "-write center.X", "-write right.X", "-write all X", "-change center", "-change window", "-change skew", "-read cursor 2", "-read cursor 1", "-read cursor 0", "-read all cursors", "-reset", "-read plot scale", "-set y to middle", "-Q: center.Y is visible", "-Q: window is visible", "-parse center.Y", "-right left from center", "-left move", "-right move", "-set center.Y", "-empty", "-set cursors to default", "-check", "-write center.Y", "-copy cursor 1", "-copy cursor 0", "-copy cursor 2", "move right", "move left", "shrink", "broaden", "skew up", "skew down", "-write plot scale", "zoom X", "change cen&win"]
            n148 = Unbundle By Name(w387) -> ("skew"=w388:dbl)
            n149 = Add(x=0.1, y=w388) -> (x+y=w385:dbl)
            n150 = call "Q -- check range -- i -- real.vi"("upper"=1, "lower"=-1, "number"=w385) -> ("number in range"=w382:dbl)  [unwired: 6 in, 2 out]
            n151 = Bundle By Name(cluster=w387, "skew"=w382) -> (w389:T1)
            n152 = call "cursor window action stack.vi"("stack action"=stack_action_--_control."push", "action list"=w393, "command stack"=w391) -> ("command stack out"=w390:T3[])  [unwired: 6 in, 2 out]
          }
        }
      }
      frame "skew down" {
        n153 = Unbundle By Name(w395) -> ("kind"=w394:enum16{"symmetric", "skewed", "fancy"})
        n154 = case shown="\"skewed\"" w394 {
          tunnel: w400 -> [w402 w413]
          tunnel: [w402 w412] -> w399
          tunnel: [w401 w411] -> w398
          tunnel: w395 -> [w401 w410]
          frame "symmetric", Default {
          }
          frame "skewed" {
            w405 = T3[] [enum."-change skew", enum."-read plot scale", enum."-set center.Y", enum."-write right.X", enum."-write left.X", enum."-write center.Y"] items=["balance", "h. offset change", "cursor moves", "change center", "change window", "init", "check", "reset", "set y to middle", "idle", "-write all Y", "-write left.X", "-write center.X", "-write right.X", "-write all X", "-change center", "-change window", "-change skew", "-read cursor 2", "-read cursor 1", "-read cursor 0", "-read all cursors", "-reset", "-read plot scale", "-set y to middle", "-Q: center.Y is visible", "-Q: window is visible", "-parse center.Y", "-right left from center", "-left move", "-right move", "-set center.Y", "-empty", "-set cursors to default", "-check", "-write center.Y", "-copy cursor 1", "-copy cursor 0", "-copy cursor 2", "move right", "move left", "shrink", "broaden", "skew up", "skew down", "-write plot scale", "zoom X", "change cen&win"]
            n155 = Unbundle By Name(w410) -> ("skew"=w404:dbl)
            n156 = Subtract(x=w404, y=0.1) -> (x-y=w409:dbl)
            n157 = call "Q -- check range -- i -- real.vi"("upper"=1, "lower"=-1, "number"=w409) -> ("number in range"=w406:dbl)  [unwired: 6 in, 2 out]
            n158 = Bundle By Name(cluster=w410, "skew"=w406) -> (w411:T1)
            n159 = call "cursor window action stack.vi"("stack action"=stack_action_--_control."push", "action list"=w405, "command stack"=w413) -> ("command stack out"=w412:T3[])  [unwired: 6 in, 2 out]
          }
        }
      }
      frame "-Q: window is visible" {
        n160 = Unbundle By Name(w425) -> ("scale.x.min"=w417:dbl, "scale.x.max"=w416:dbl, "scale.x.center"=w420:dbl, "scale.x.range"=w415:dbl)  [unwired: 1 out]
        n161 = Unbundle By Name(w419) -> ("center"=w424:dbl)
        n162 = call "Q -- check range -- i -- real.vi"("upper"=w416, "lower"=w417, "number"=w424) -> ("selector"=w423:T8)  [unwired: 6 in, 2 out]
        n163 = case shown="\"not a number\", \"above\", \"below\", Default" w423 {
          tunnel: w422 -> [w432 w457]
          tunnel: [w431 w455] -> w421
          tunnel: w419 -> [w430 w454]
          tunnel: w420 -> [_ w453]
          tunnel: [w428 w452] -> w418
          tunnel: w417 -> [w438 _]
          tunnel: w416 -> [w437 _]
          tunnel: w415 -> [w429 _]
          frame "in range" {
            n164 = Unbundle By Name(w430) -> ("left"=w440:dbl, "right"=w439:dbl)
            n165 = call "Q -- check range -- i -- real.vi"("upper"=w437, "lower"=w438, "number"=w440) -> ("in range?"=w436:bool)  [unwired: 6 in, 2 out]
            n166 = call "Q -- check range -- i -- real.vi"("upper"=w437, "lower"=w438, "number"=w439) -> ("in range?"=w435:bool)  [unwired: 6 in, 2 out]
            n167 = Not(x=w436) -> (.not. x?=w434:bool)
            n168 = Not(x=w435) -> (.not. x?=w433:bool)
            n169 = And(x=w434, y=w433) -> (x .and. y?=w427:bool)
            n170 = case shown="True" w427 {
              tunnel: w432 -> [w442 w449]
              tunnel: [w442 w448] -> w431
              tunnel: w430 -> [w441 w447]
              tunnel: w429 -> [_ w445]
              tunnel: [w441 w443] -> w428
              frame False {
              }
              frame True {
                w451 = T3[] [enum."-change window", enum."-write left.X", enum."-write right.X"] items=["balance", "h. offset change", "cursor moves", "change center", "change window", "init", "check", "reset", "set y to middle", "idle", "-write all Y", "-write left.X", "-write center.X", "-write right.X", "-write all X", "-change center", "-change window", "-change skew", "-read cursor 2", "-read cursor 1", "-read cursor 0", "-read all cursors", "-reset", "-read plot scale", "-set y to middle", "-Q: center.Y is visible", "-Q: window is visible", "-parse center.Y", "-right left from center", "-left move", "-right move", "-set center.Y", "-empty", "-set cursors to default", "-check", "-write center.Y", "-copy cursor 1", "-copy cursor 0", "-copy cursor 2", "move right", "move left", "shrink", "broaden", "skew up", "skew down", "-write plot scale", "zoom X", "change cen&win"]
                n171 = Unbundle By Name(w447) -> ("default window frac"=w446:dbl)
                n172 = Multiply(x=w446, y=w445) -> (x*y=w444:dbl)
                n173 = Bundle By Name(cluster=w447, "window"=w444) -> (w443:T1)
                n174 = call "cursor window action stack.vi"("stack action"=stack_action_--_control."push", "action list"=w451, "command stack"=w449) -> ("command stack out"=w448:T3[])  [unwired: 6 in, 2 out]
              }
            }
          }
          frame "not a number", "above", "below", Default {
            w458 = T3[] [enum."-change center", enum."-write all X", enum."-Q: window is visible"] items=["balance", "h. offset change", "cursor moves", "change center", "change window", "init", "check", "reset", "set y to middle", "idle", "-write all Y", "-write left.X", "-write center.X", "-write right.X", "-write all X", "-change center", "-change window", "-change skew", "-read cursor 2", "-read cursor 1", "-read cursor 0", "-read all cursors", "-reset", "-read plot scale", "-set y to middle", "-Q: center.Y is visible", "-Q: window is visible", "-parse center.Y", "-right left from center", "-left move", "-right move", "-set center.Y", "-empty", "-set cursors to default", "-check", "-write center.Y", "-copy cursor 1", "-copy cursor 0", "-copy cursor 2", "move right", "move left", "shrink", "broaden", "skew up", "skew down", "-write plot scale", "zoom X", "change cen&win"]
            n175 = Bundle By Name(cluster=w454, "center"=w453) -> (w452:T1)
            n176 = call "cursor window action stack.vi"("stack action"=stack_action_--_control."push", "action list"=w458, "command stack"=w457) -> ("command stack out"=w455:T3[])  [unwired: 6 in, 2 out]
          }
        }
      }
    }
    n177 = call "cursor window action stack.vi"("stack action"=stack_action_--_control."check", "command stack"=w28) -> ("stack is empty ?"=w26:bool, "command stack out"=w27:T3[])  [unwired: 7 in, 1 out]
  }
  "cursor window out" <- w1
